vi "Register to Discovery Service.vi"(8 "error in":errorcluster, 10 "PortNumber":i32, 11 "gRPC ID":T2) -> (0 "error out":errorcluster, 2 "Response Data":T1, 3 "gRPC ID out":T2)   [LabVIEW 2020, in "Line Regulation.lvlib"]
uses:
  Line Regulation.lvlib
  <vilib>/gRPC/LabVIEW gRPC Library/Server API/typeDefs/grpcId.ctl
  <vilib>/TAF/Discovery Client/RPC Messages/NIMeasurementServices_RegisterServiceResponse.ctl
  <vilib>/TAF/Discovery Client/RPC Messages/NIMeasurementServices_RegisterServiceRequest.ctl
  <vilib>/TAF/Discovery Client/RPC Messages/NIMeasurementServices_ServiceDescriptor.ctl
  <vilib>/TAF/Discovery Client/RPC Messages/NIMeasurementServices_ServiceLocation.ctl
  <vilib>/TAF/Discovery Client/Discovery_client.lvlib
  <vilib>/gRPC/LabVIEW gRPC Library/gprc-lvsupport-release.lvlib
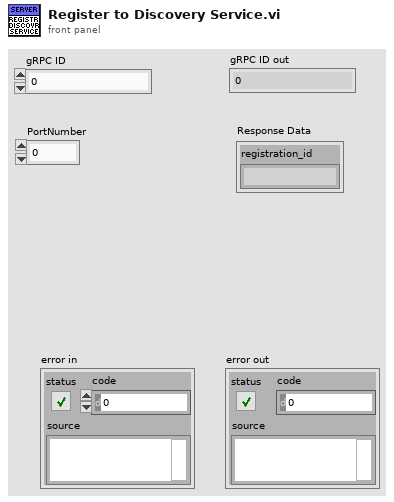
[diagram p1: front panel]
types:
  T1 = typedef "Discovery_client.lvlib/NIMeasurementServices_RegisterServiceResponse.ctl" = cluster{"registration_id":string}
  T2 = typedef "gprc-lvsupport-release.lvlib/grpcId.ctl" = u64
  T3 = typedef "Discovery_client.lvlib/NIMeasurementServices_RegisterServiceRequest.ctl" = cluster{"service_description":T4, "provided_services":string[], "location":T5}
  T4 = typedef "Discovery_client.lvlib/NIMeasurementServices_ServiceDescriptor.ctl" = cluster{"service_id":string, "name":string, "description_url":string, "service_class":string}
  T5 = typedef "Discovery_client.lvlib/NIMeasurementServices_ServiceLocation.ctl" = cluster{"location":string, "optimal_route":string, "insecure_port":string, "ssl_authenticated_port":string}
  T6 = typedef "Line Regulation.lvlib/ni_measurements_v1_MeasurementDetails.ctl" = cluster{"display_name":string, "version":string, "measurement_type":string, "product_type":string}
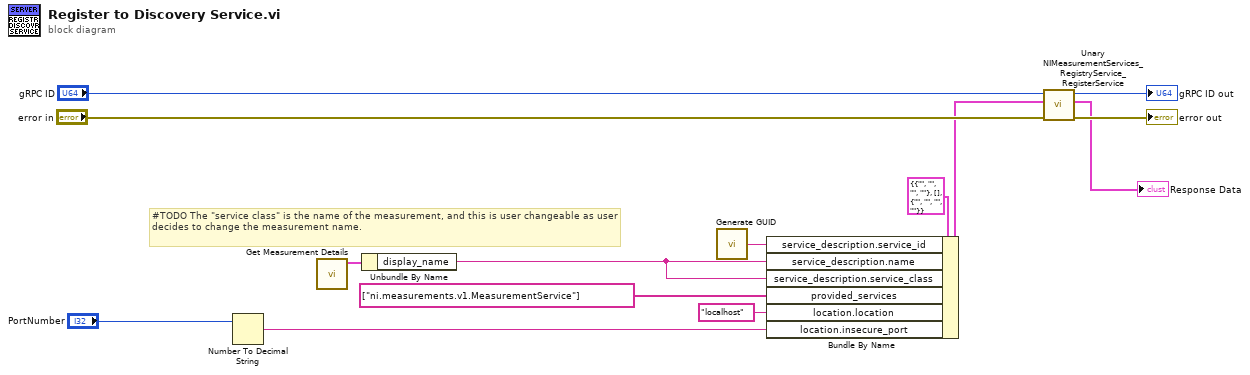
[diagram p0: block diagram]
diagram:
  # "#TODO The \"service class\" is the name of the measurement, and this is user changeable as user decides to change the measurement name."
  n1 = Number To Decimal String(number="PortNumber") -> (decimal integer string=w14:string)  [unwired: 1 in]
  n2 = call "Get Measurement Details.vi"() -> ("measurement_details"=w10:T6)  [unwired: 10 in, 1 out]
  n3 = Unbundle By Name(w10) -> ("display_name"=w9:string)
  n4 = call "Generate GUID.vi"() -> ("ToString"=w11:string)  [unwired: 5 in]
  n5 = Bundle By Name(cluster=T3 {"service_description"={"service_id"="", "name"="", "description_url"="", "service_class"=""}, "provided_services"=[], "location"={"location"="", "optimal_route"="", "insecure_port"="", "ssl_authenticated_port"=""}} ("Request Data"), "service_description.service_id"=w11, "service_description.name"=w9, "service_description.service_class"=w9, "provided_services"=string[] ["ni.measurements.v1.MeasurementService"], "location.location"="localhost", "location.insecure_port"=w14) -> (w3:T3)
  n6 = call <vilib>:"Unary NIMeasurementServices_RegistryService_RegisterService.vi"("error in"="error in", "Request Data"=w3, "gRPC ID"="gRPC ID") -> ("error out"=→"error out":errorcluster, "Response Data"=→"Response Data":T1, "gRPC ID out"=→"gRPC ID out":T2)  [unwired: 6 in]
